vi "Pre Launch Init.vi"(11 "Instrument in":refnum<class "Instrument.lvclass">) -> (0 "error out":errorcluster, 3 "Instrument out":refnum<class "Instrument.lvclass">)   [LabVIEW 2015, in "Item Actor.lvlib" / "Instrument.lvclass"]
doc: "(<B>Filename</B>: Actor Framework.lvlib:Actor.lvclass:Pre Launch Init.vi)\n\nDefines behavior that occurs after the Launch Nested Actor method is invoked but before the actor's Actor Core method begins running.\n\nBy default, this method does nothing. A descendant class may override it to define behavior."
uses:
  Instrument.lvclass
  Generic Item/Generic Item.lvclass
  Instrument.lvclass/Instrument.ctl
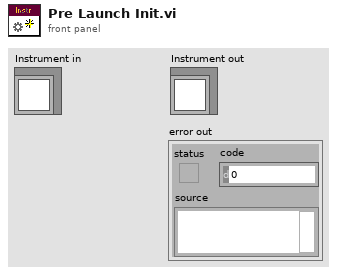
[diagram p1: front panel]
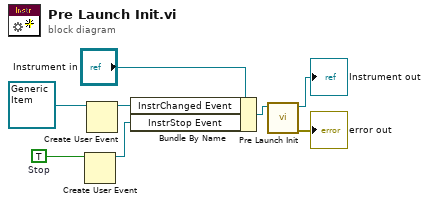
[diagram p0: block diagram]
diagram:
  w2 = TRUE  # Stop
  n1 = Create User Event(user event datatype=w2) -> (user event=w1:refnum<user-event>)  [unwired: 1 in, 1 out]
  n2 = Create User Event(user event datatype=refnum<class "Generic Item.lvclass"> refnum ("Item Actor.lvlib:Generic Item.lvclass")) -> (user event=w4:refnum<user-event>)  [unwired: 1 in, 1 out]
  n3 = Bundle By Name(cluster="Instrument in", "InstrChanged Event"=w4, "InstrStop Event"=w1) -> (w5:refnum<class "Instrument.lvclass">)
  n4 = call-parent "Pre Launch Init.vi"("Actor in"=w5) -> ("error out"=→"error out":errorcluster, "Actor out"=→"Instrument out":refnum<class "Instrument.lvclass">)  [unwired: 9 in]
